vi "Convert input voltages.vi"(8 "error in (no error)":errorcluster, 11 "BMC in":refnum<class "BMC.lvclass">) -> (0 "error out":errorcluster, 2 "Command Array":i16[](array[numeric]), 3 "BMC out":refnum<class "BMC.lvclass">)   [LabVIEW 2012, in "BMC.lvclass"]
uses:
  BMC.lvclass
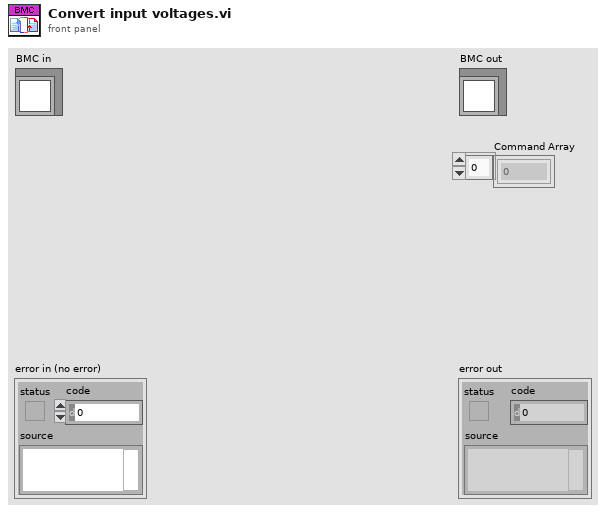
[diagram p1: front panel]
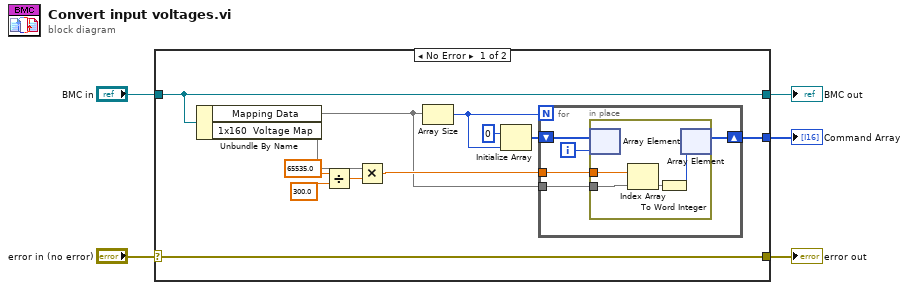
[diagram p0: block diagram]
diagram:
  n1 = case shown="No Error" "error in (no error)" {
    selector: "error in (no error)" -> [w17 w28]
    tunnel: [w17 w28] -> w4
    tunnel: [w12 w27] -> w2
    tunnel: "BMC in" -> [w12 w27]
    tunnel: [w10 _] -> w1
    frame No Error {
      n2 = Unbundle By Name(w12) -> ("Mapping Data"=w8, "1x160  Voltage Map"=w7)
      n3 = Divide(x=65535.0 ("y"), y=300.0 ("x")) -> (x/y=w6:dbl)
      n4 = Multiply(x=w7, y=w6) -> (x*y=w9:dbl)
      n5 = Array Size(array=w8) -> (size(s)=w16:i32)
      n6 = Initialize Array(i16 0 ("element"), w16) -> (w14:i16[])
      n7 = for {
        N: w16 -> [_]
        shift-right: [w20] -> w10
        shift-left: w14 -> [w22]
        tunnel: w9 -> [w21]
        tunnel: w8 -> [w18]
        i -> [w19]
        n8 = in-place {
          in-place-border: w21 -> [w25]
          in-place-border: w18 -> [w26]
          n9 = in-place-array #1(w22, w19) -> ()  [unwired: 1 out]
          n10 = Index Array(array=w25, index=w26) -> (element=w24)
          n11 = To Word Integer(number=w24) -> (16bit integer=w23:i16)
          n12 = in-place-array #1(w23) -> (w20:i16[])  [unwired: 1 out]
        }
      }
    }
    frame Error {
    }
  }
  "error out" <- w4
  "BMC out" <- w2
  "Command Array" <- w1
